vi "Set Port Status.vi"(8 "error in (no error)":errorcluster, 9 "Value":string, 10 "Port":dbl, 11 "object in":refnum<class "Simulado.lvclass">) -> (0 "error out":errorcluster, 3 "object out":refnum<class "Simulado.lvclass">)   [LabVIEW 2020, in "Simulado.lvclass"]
uses:
  Simulado.lvclass
  Abstract/Serial Device/Serial Device.lvclass
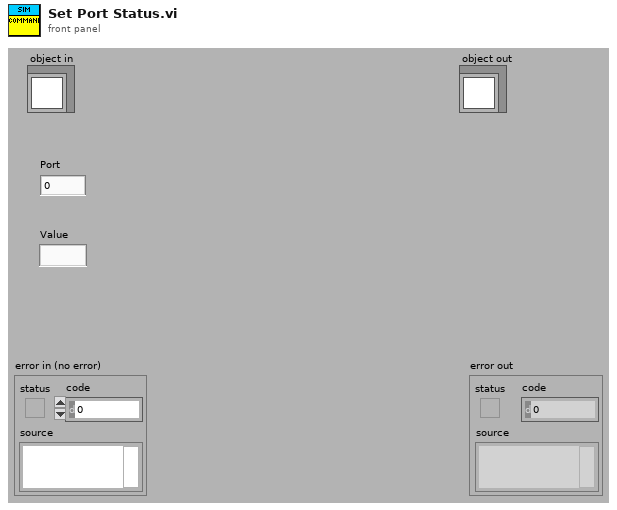
[diagram p1: front panel]
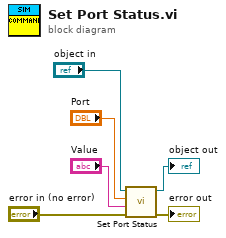
[diagram p0: block diagram]
diagram:
  n1 = call-parent "Set Port Status.vi"("error in (no error)"="error in (no error)", "Value"="Value", "Port"="Port", "object in"="object in") -> ("error out"=→"error out":errorcluster, "object out"=→"object out":refnum<class "Simulado.lvclass">)  [unwired: 6 in]
